vi "Float_TO_WORD.vi"(11 "FLOAT":sgl) -> (2 "second_Word":u16, 3 "first_Word":u16)   [LabVIEW 2023, in "Drive.lvlib"]
uses:
  Drive.lvlib
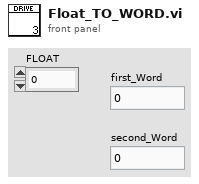
[diagram p1: front panel]
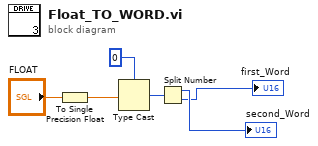
[diagram p0: block diagram]
diagram:
  n1 = To Single Precision Float(number="FLOAT") -> (single precision float=w5:sgl)
  n2 = Type Cast(type=u32 0 ("(hi.lo)"), x=w5) -> (*(type *) &x=w4:u32)
  n3 = Split Number(x=w4) -> (hi(x)=→"second_Word":u16, lo(x)=→"first_Word":u16)
